vi "SHOOT.vi"(10 "argv":string[](array[string]), 11 "args":u8) -> ()   [LabVIEW 2015]
uses:
  Team Code/Robot Global Data.vi
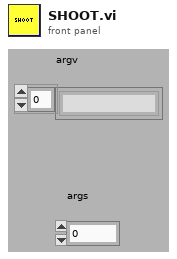
[diagram p1: front panel]
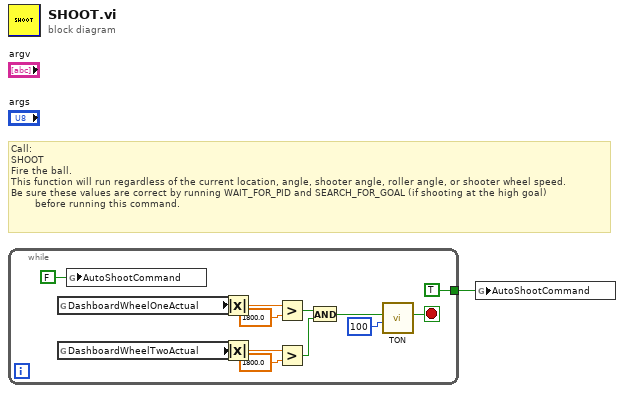
[diagram p0: block diagram]
diagram:
  # "Call:\nSHOOT\nFire the ball.\nThis function will run regardless of the current location, angle, shooter angle, roller angle, or shooter wheel speed.\nBe sure these values are correct by running WAIT_FOR_PID and SEARCH_FOR_GOAL (if shooting at the high goal)\n        before running this command."
  n1 = while {
    tunnel: [TRUE] -> w1
    stop <- w11 stop-if-true
    n2 = global read "Robot Global Data.vi" "DashboardWheelOneActual"() -> (w9:dbl)
    n3 = global read "Robot Global Data.vi" "DashboardWheelTwoActual"() -> (w8:dbl)
    n4 = global write "Robot Global Data.vi" "AutoShootCommand"(FALSE ("AutoArmControl")) -> ()
    n5 = Absolute Value(x=w9) -> (abs(x)=w3:dbl)
    n6 = Absolute Value(x=w8) -> (abs(x)=w2:dbl)
    n7 = Greater?(x=w3, y=1800.0) -> (0:w4:bool)
    n8 = Greater?(x=w2, y=1800.0) -> (0:w5:bool)
    n9 = And(x=w4, y=w5) -> (x .and. y?=w12:bool)
    n10 = call "TON.vi"("Delay (ms)"=u32 100, "Input"=w12) -> ("Output"=w11:bool)  [unwired: 9 in]
  }
  n11 = global write "Robot Global Data.vi" "AutoShootCommand"(w1) -> ()
